vi "GreenHouse.vi"() -> ()   [LabVIEW 2014]
panel:
  out "sensor- if block":bool
  out "light":bool
  in  "door close limit":bool
  in  "door open limit":bool
  out "motor":bool
  in  "Temperature":dbl(slide) scale=-100.0..100.0
  in  "stop":bool
  out "current differ from min 2":dbl
  out "current differ from max 2":dbl
  out "current differ from min":dbl
  out "current differ from max":dbl
  out "water":bool
  out "Heater":bool
  out "Open":bool
  in  "maximum temp":dbl
  in  "minimum temp":dbl
  in  "maximum humidity":dbl
  in  "minimum humidity":dbl
  in  "Humidity":dbl(slide) scale=0.0..100.0
  # "User input"
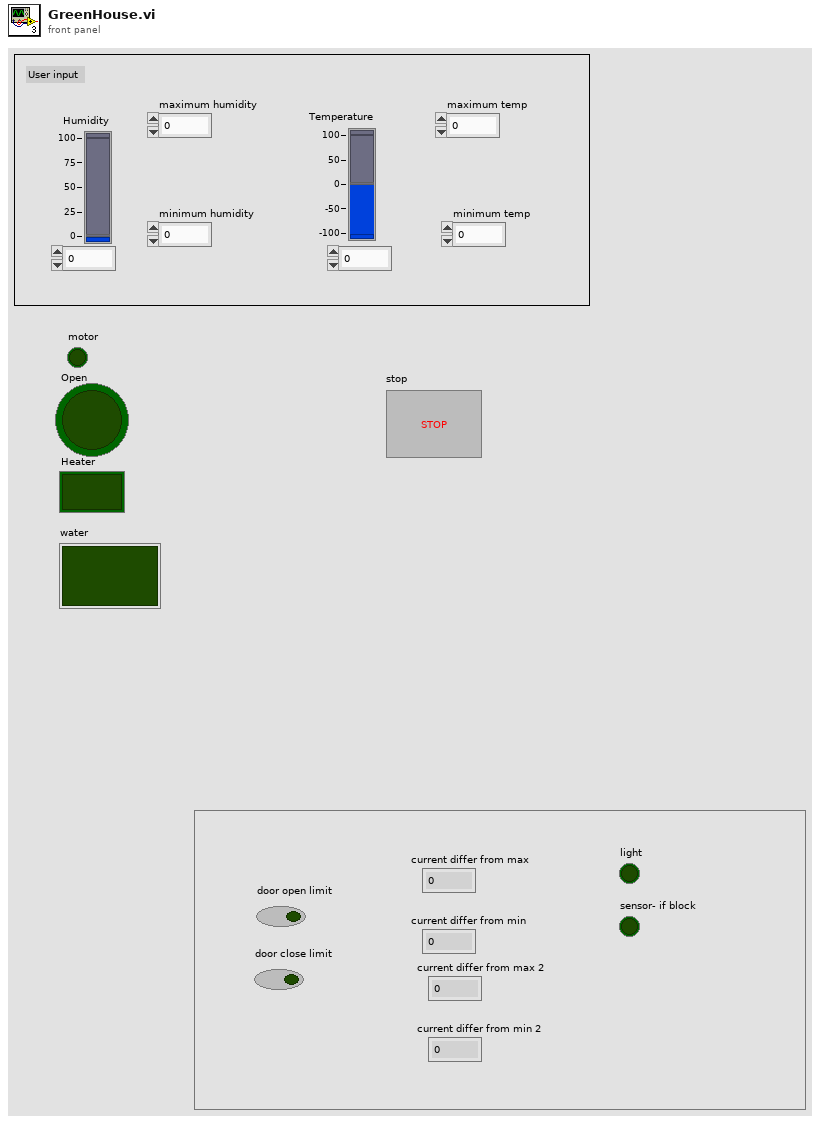
[diagram p1: front panel]
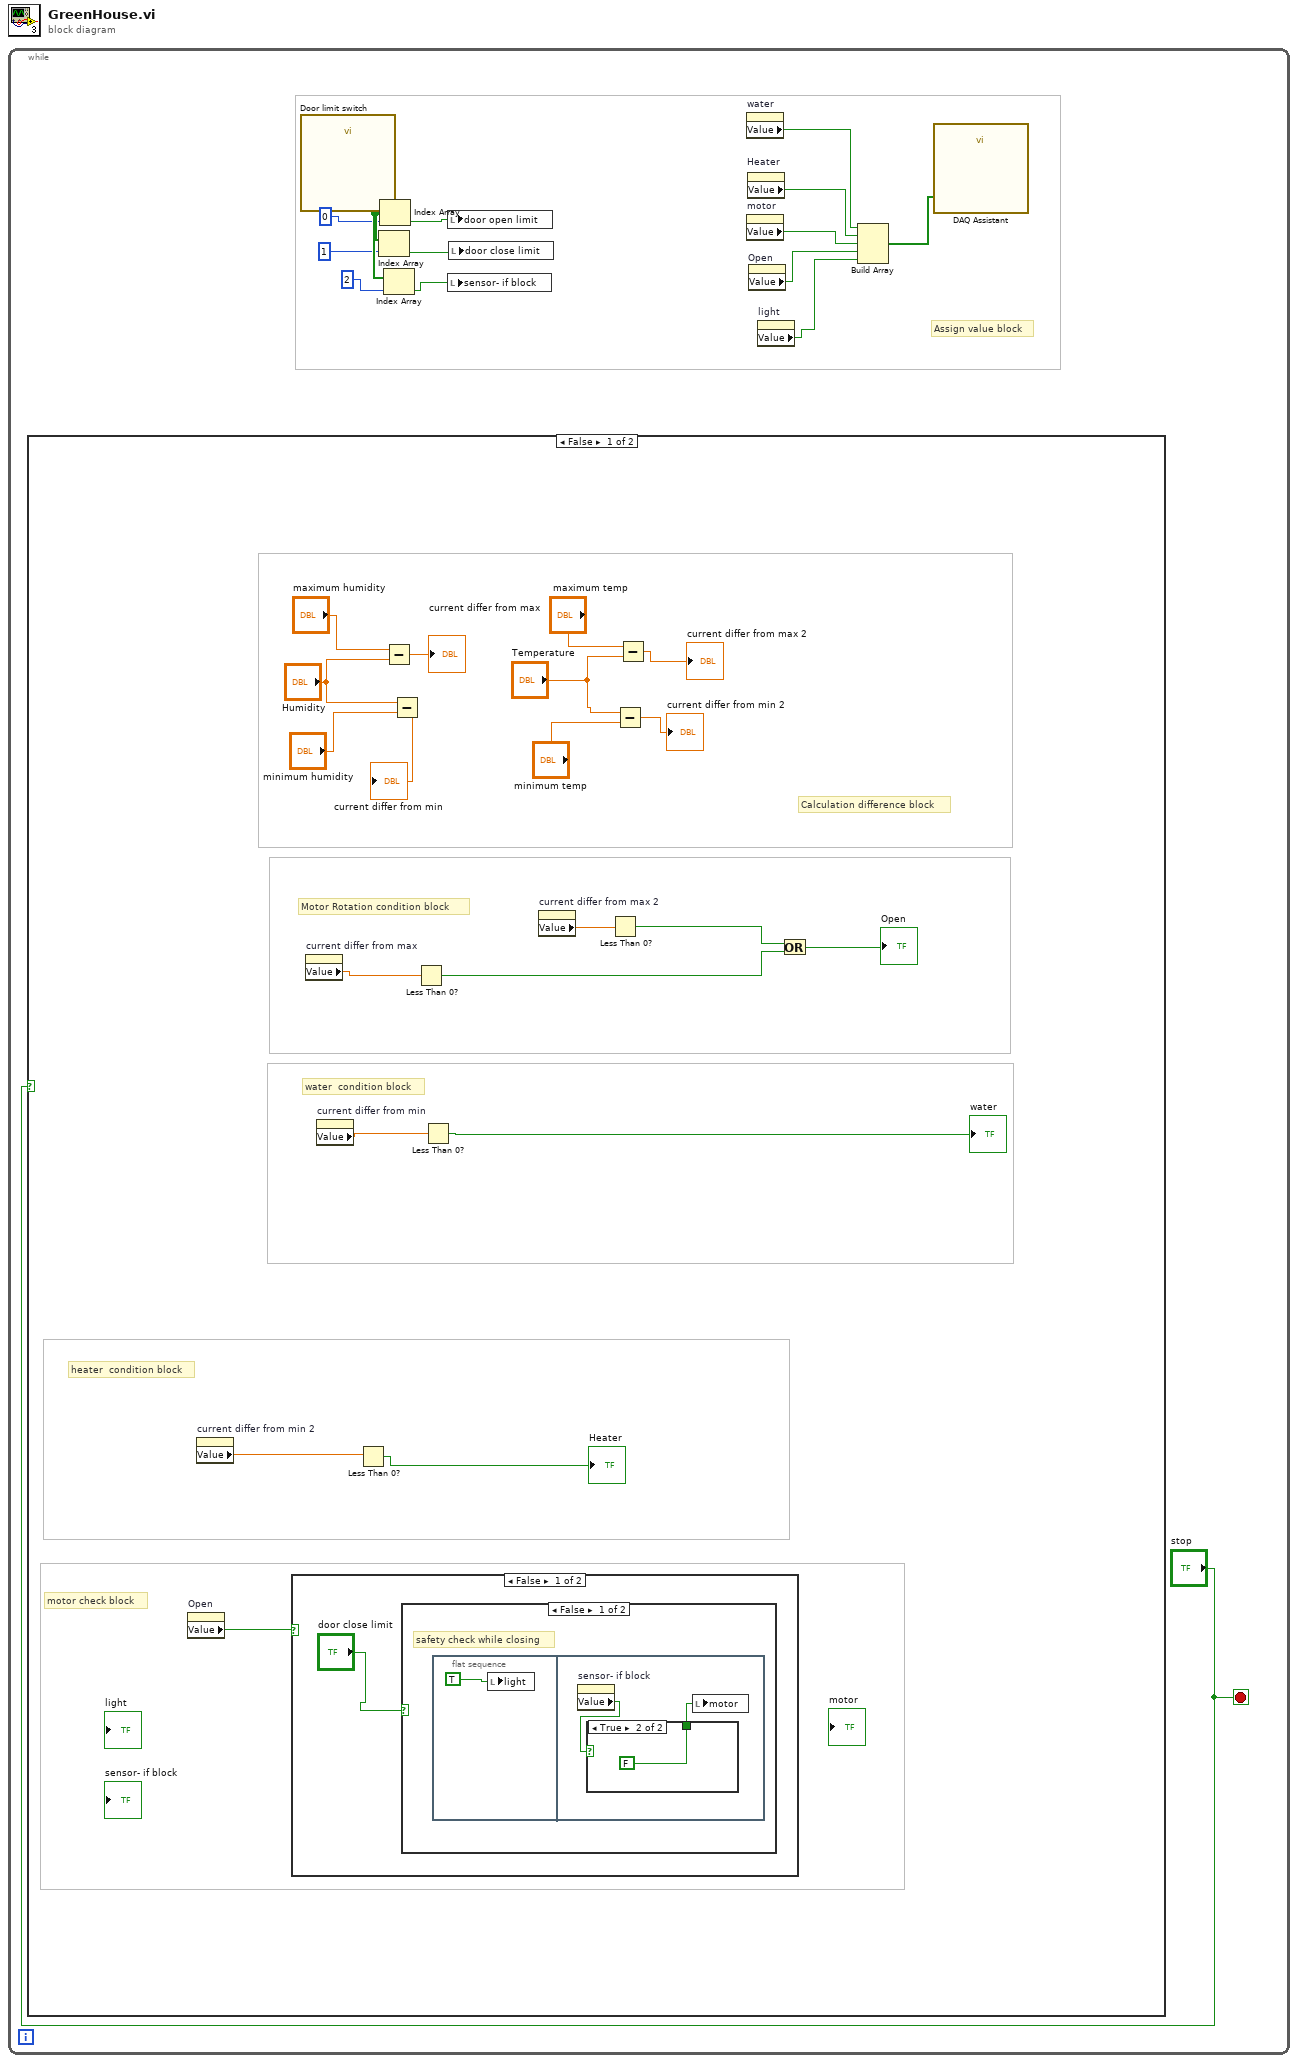
[diagram p0: block diagram]
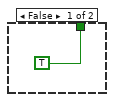
[diagram p2: hidden frame]
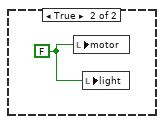
[diagram p3: hidden frame]
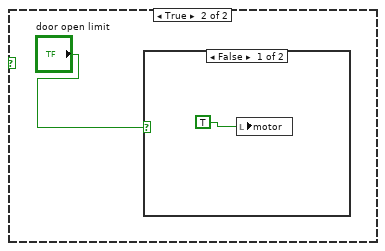
[diagram p4: hidden frame]
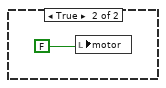
[diagram p5: hidden frame]
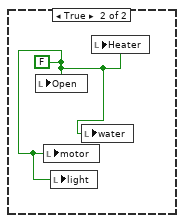
[diagram p6: hidden frame]
diagram:
  n1 = while {
    stop <- "stop" stop-if-true
    # "Assign value block"
    n2 = case shown="False" "stop" {
      frame False {
        # "Calculation difference block"
        # "motor check block"
        # "heater  condition block"
        # "water  condition block"
        # "Motor Rotation condition block"
        n3 = property on="Open" class="Bool (strict)"() -> ("Value"=w17:bool)  [unwired: 2 in, 2 out]
        n4 = property on="current differ from min 2" class="DigNum (strict)"() -> ("Value"=w22:dbl)  [unwired: 2 in, 2 out]
        n5 = case shown="False" w17 {
          frame False {
            n6 = case shown="False" "door close limit" {
              frame False {
                # "safety check while closing"
                n7 = flat-sequence {
                  frame #0 {
                    n8 = local write "light"(TRUE) -> ()
                  }
                  frame #1 {
                    n9 = property on="sensor- if block" class="Bool (strict)"() -> ("Value"=w38:bool)  [unwired: 2 in, 2 out]
                    n10 = case shown="True" w38 {
                      tunnel: [TRUE FALSE] -> w37
                      frame False {
                      }
                      frame True {
                      }
                    }
                    n11 = local write "motor"(w37) -> ()
                  }
                }
              }
              frame True {
                w41 = FALSE
                n12 = local write "motor"(w41) -> ()
                n13 = local write "light"(w41) -> ()
              }
            }
          }
          frame True {
            n14 = case shown="False" "door open limit" {
              frame False {
                n15 = local write "motor"(TRUE) -> ()
              }
              frame True {
                n16 = local write "motor"(FALSE) -> ()
              }
            }
          }
        }
        n17 = property on="current differ from max" class="DigNum (strict)"() -> ("Value"=w33:dbl)  [unwired: 2 in, 2 out]
        n18 = property on="current differ from min" class="DigNum (strict)"() -> ("Value"=w28:dbl)  [unwired: 2 in, 2 out]
        n19 = Less Than 0?(x=w22) -> (x < 0?=→"Heater":bool)
        n20 = Subtract(x="maximum humidity", y="Humidity") -> (x-y=→"current differ from max":dbl)
        n21 = Subtract(x="Humidity", y="minimum humidity") -> (x-y=→"current differ from min":dbl)
        n22 = Less Than 0?(x=w33) -> (x < 0?=w15:bool)
        n23 = Less Than 0?(x=w28) -> (x < 0?=→"water":bool)
        n24 = property on="current differ from max 2" class="DigNum (strict)"() -> ("Value"=w19:dbl)  [unwired: 2 in, 2 out]
        n25 = Less Than 0?(x=w19) -> (x < 0?=w16:bool)
        n26 = Subtract(x="Temperature", y="minimum temp") -> (x-y=→"current differ from min 2":dbl)
        n27 = Subtract(x="maximum temp", y="Temperature") -> (x-y=→"current differ from max 2":dbl)
        n28 = Or(x=w16, y=w15) -> (x .or. y?=→"Open":bool)
      }
      frame True {
        w45 = FALSE
        n29 = local write "Open"(w45) -> ()
        n30 = local write "motor"(w45) -> ()
        n31 = local write "light"(w45) -> ()
        n32 = local write "water"(w45) -> ()
        n33 = local write "Heater"(w45) -> ()
      }
    }
    n34 = call "Door limit switch"() -> ("data"=w7:bool[])  [unwired: 17 in, 2 out]
    n35 = Index Array(array=w7, index=1) -> (element=w8:bool)
    n36 = Index Array(array=w7, index=0) -> (element=w2:bool)
    n37 = Index Array(array=w7, index=2) -> (element=w5:bool)
    n38 = local write "door open limit"(w2) -> ()
    n39 = local write "sensor- if block"(w5) -> ()
    n40 = local write "door close limit"(w8) -> ()
    n41 = property on="water" class="Bool (strict)"() -> ("Value"=w9:bool)  [unwired: 2 in, 2 out]
    n42 = property on="motor" class="Bool (strict)"() -> ("Value"=w11:bool)  [unwired: 2 in, 2 out]
    n43 = property on="Heater" class="Bool (strict)"() -> ("Value"=w10:bool)  [unwired: 2 in, 2 out]
    n44 = property on="Open" class="Bool (strict)"() -> ("Value"=w12:bool)  [unwired: 2 in, 2 out]
    n45 = property on="light" class="Bool (strict)"() -> ("Value"=w13:bool)  [unwired: 2 in, 2 out]
    n46 = Build Array(w9, w10, w11, w12, w13) -> (w14:bool[])
    n47 = call "DAQ Assistant"("data"=w14) -> ()  [unwired: 17 in, 2 out]
  }
